vi "board parameters.vi"() -> ()   [LabVIEW 2015]
uses:
  dio64/labview(m)/dio64_32.llb/DIO64 Out Config Control.ctl
  dio64/labview(m)/dio64_32.llb/DIO64 clock control.ctl
  dio64/labview(m)/dio64_32.llb/DIO64 start trig.ctl
  dio64/labview(m)/dio64_32.llb/DIO64 stop trig.ctl
panel:
  in  "Config Control":T1 {"#transitions" format="%.0x"; "repetitions" format="%.0x"; "DAQ clock modulo" format="%.0x"}
  in  "Data to the board":u32[][](array[numeric])
  in  "Mask":u16[](array[numeric])=[65535] format="%.0x"
  in  "# of ports":u16=4
  in  "Initial data":u16[][](array[numeric])=[[0, 6, 1]] format="%.0b"
  in  "Clock Frequency":dbl=1000000.0 format="%.2f"
  in  "Base I/O":u16=384 format="%.0x"
  in  "Board":u16
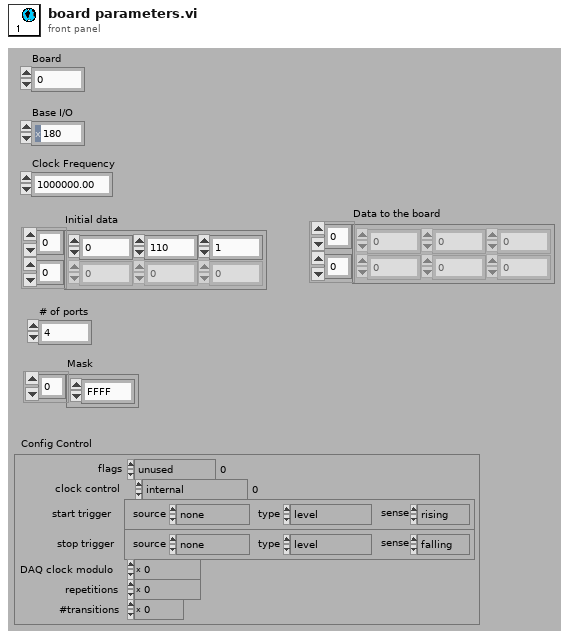
[diagram p1: front panel]
types:
  T1 = typedef "DIO64 Out Config Control.ctl" = cluster{"flags":enum16{"unused"}, "clock control":T2, "start trigger":T3, "stop trigger":T4, "DAQ clock modulo":u32, "repetitions":u32, "#transitions":u16}
  T2 = typedef "DIO64 clock control.ctl" = enum16{"internal", "external", "trig 0", "OCXO"}
  T3 = typedef "DIO64 start trig.ctl" = cluster{"source":enum16{"none", "internal", "external", "trig 2", "PXI Star"}, "type":enum16{"level", "edge", "edge to edge"}, "sense":enum16{"rising", "falling"}}
  T4 = typedef "DIO64 stop trig.ctl" = cluster{"source":enum16{"none", "internal", "external", "trig 3 in", "output FIFO"}, "type":enum16{"level", "edge"}, "sense":enum16{"falling", "rising"}}
diagram:
